vi "write_msg_to_log.vi"(10 "error_msg_to_log":string, 11 "Error in":refnum<class "Error.lvclass">) -> (3 "Error out":refnum<class "Error.lvclass">)   [LabVIEW 2023, in "Error Handling Interface.lvlib" / "Error.lvclass"]
uses:
  Error.lvclass
  Error.lvclass/Error.ctl
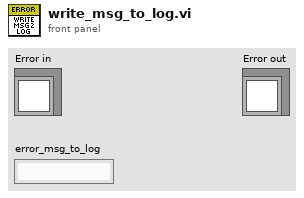
[diagram p1: front panel]
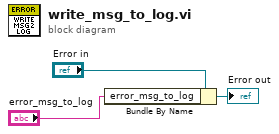
[diagram p0: block diagram]
diagram:
  n1 = Bundle By Name(cluster="Error in", "error_msg_to_log"="error_msg_to_log") -> (→"Error out":refnum<class "Error.lvclass">)
